vi "FPGA Main_4Modules.vi"() -> ()   [LabVIEW 2015]
doc: "This FPGA Main VI contains a control loop running in parallel with an RT watchdog loop.\n- The Control Loop performs control calculations on four input channels in parallel, and outputs the results to four output channels.\n- The RT Watchdog Loop checks for a periodic 'pet' from the RT Main VI to ensure communications between RT and FPGA are maintained."
uses:
  <vilib>/eio/EIONode/EIONode.xnode
  <vilib>/rvi/eio/common/nirviEmuTemplateMethod_errors.vi
  <vilib>/eio/EIOPropertyNode/EIOPropertyNode.xnode
  <vilib>/rvi/DataTransferAndStorage/Container/XNode/niFpgaContainer.xnode
  <vilib>/rvi/eio/common/nirviEmuTemplatePropertyGet_errors.vi
  <vilib>/rvi/eio/common/nirviEmuTemplatePropertyGet_noerrors.vi
  <vilib>/rvi/eio/common/nirviEmuTemplatePropertySet_errors.vi
  <vilib>/rvi/eio/common/nirviEmuTemplatePropertySet_noerrors.vi
  <vilib>/rvi/interface/RandomDataEmulation/nirviRandomDataFpgaReadWriteTemplate.vi
  <vilib>/LabVIEW Targets/FPGA/cRIO/shared/nicrio_ModuleControls/nicrio_cRIO-9234_DataRatesRing2.ctl
panel:
  in  "Data Rate":T1=1 items=["51.200 kS/s (NI 9234)"=1, "25.600 kS/s (NI 9234)"=2, "17.067 kS/s (NI 9234)"=3, "12.800 kS/s (NI 9234)"=4, "10.240 kS/s (NI 9234)"=5, "8.533 kS/s (NI 9234)"=6, "7.314 kS/s (NI 9234)"=7, "6.400 kS/s (NI 9234)"=8, "5.689 kS/s (NI 9234)"=9, "5.120 kS/s (NI 9234)"=10, "4.654 kS/s (NI 9234)"=11, "4.267 kS/s (NI 9234)"=12, "3.938 kS/s (NI 9234)"=13, "3.657 kS/s (NI 9234)"=14, "3.413 kS/s (NI 9234)"=15, "3.200 kS/s (NI 9234)"=16, "3.012 kS/s (NI 9234)"=17, "2.845 kS/s (NI 9234)"=18, "2.695 kS/s (NI 9234)"=19, "2.560 kS/s (NI 9234)"=20, "2.438 kS/s (NI 9234)"=21, "2.328 kS/s (NI 9234)"=22, "2.226 kS/s (NI 9234)"=23, "2.133 kS/s (NI 9234)"=24, "2.048 kS/s (NI 9234)"=25, "1.969 kS/s (NI 9234)"=26, "1.896 kS/s (NI 9234)"=27, "1.829 kS/s (NI 9234)"=28, "1.765 kS/s (NI 9234)"=29, "1.707 kS/s (NI 9234)"=30, "1.652 kS/s (NI 9234)"=31]
  out "FPGA Error":errorcluster
  out "Finished":bool
  in  "Stop":bool
  out "Module Underflow":bool
  out "DMA FIFO Full":bool
  out "Different Channel Count":bool
  out "Actual Loop Period (ticks)":u32
  out "First Read":bool
  in  "Number of Channels":i32=16
  in  "Channel Scale Array":fxp<+,24,12>[](array[numeric])=[0.0, 0.0, 0.0, 0.0, 0.0, 0.0, 0.0, 0.0, 0.0, 0.0, 0.0, 0.0, 0.0, 0.0, 0.0, 0.0]
  # "General Settings"
  # "Monitoring Values"
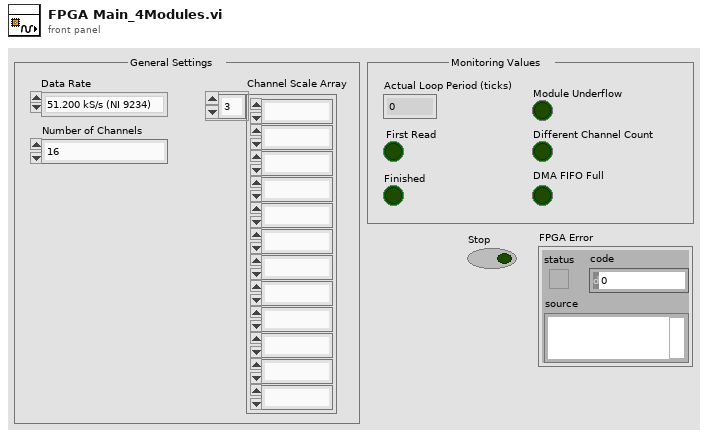
[diagram p1: front panel]
types:
  T1 = typedef "nicrio_cRIO-9234_DataRatesRing2.ctl" = u8
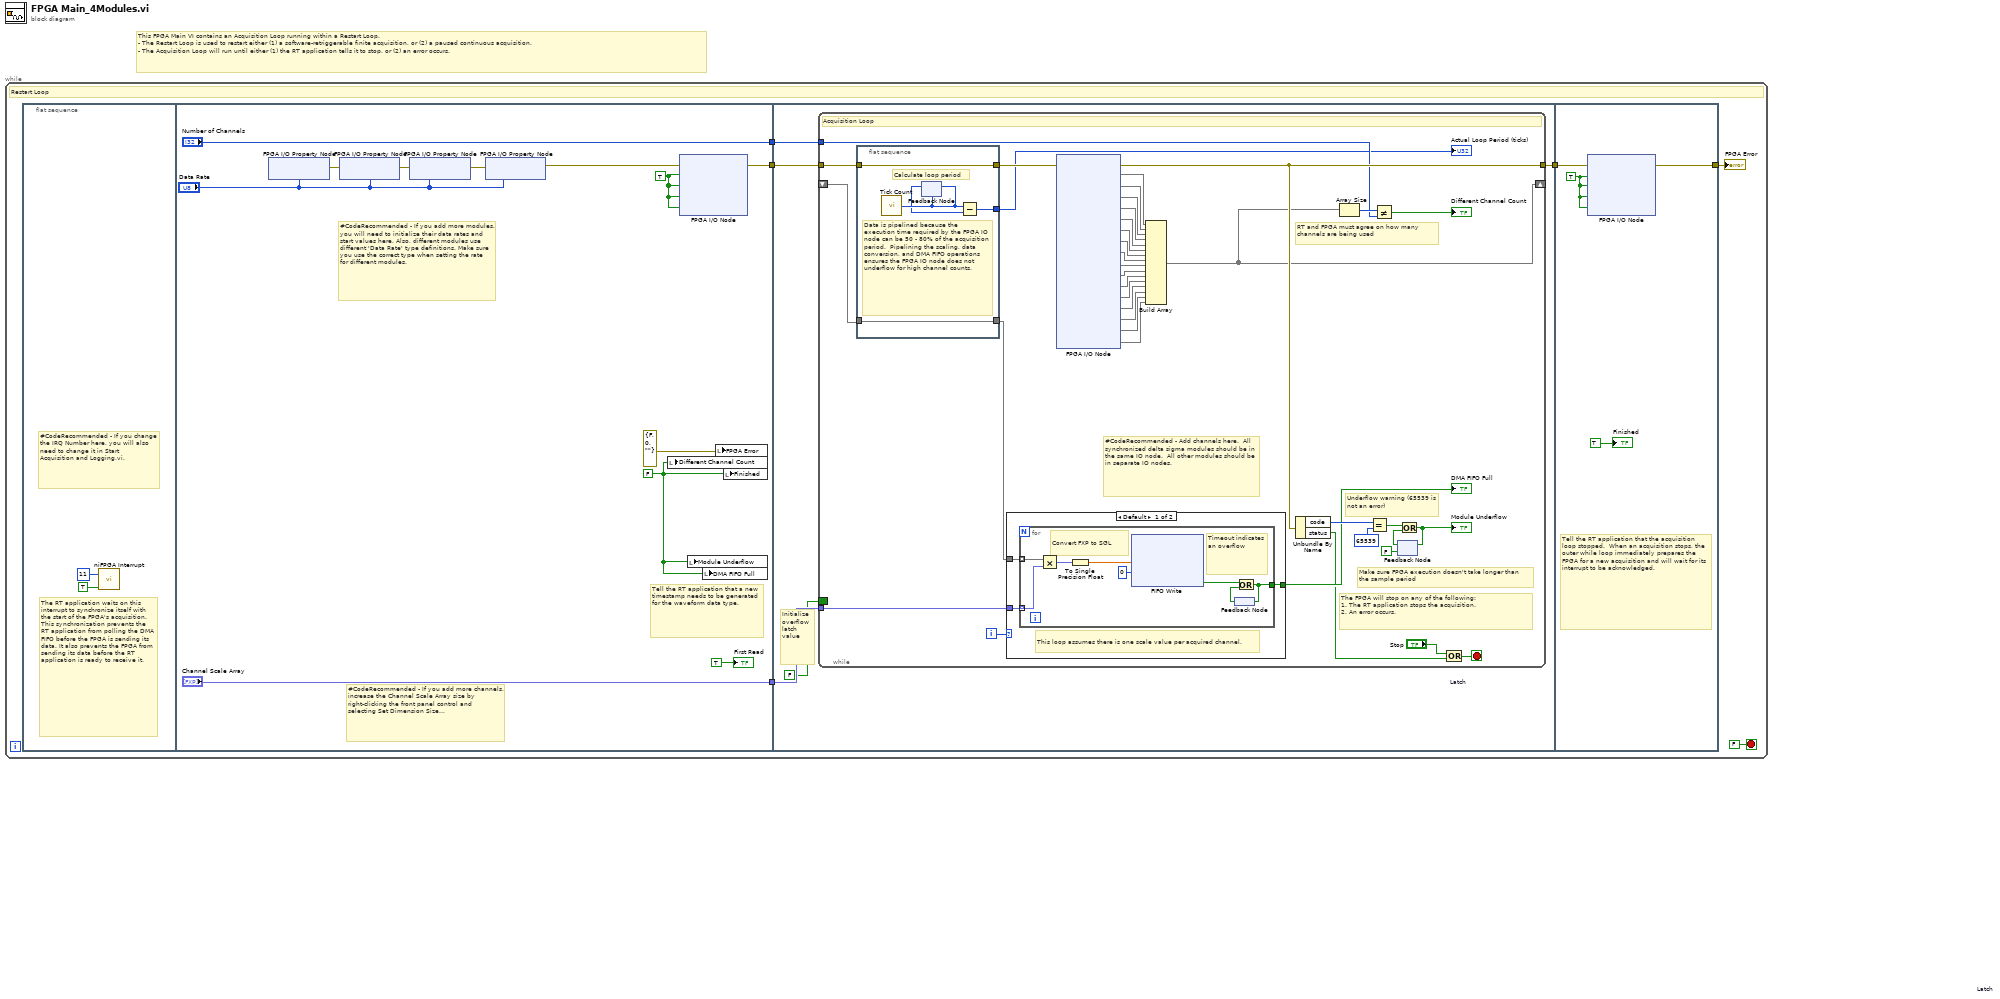
[diagram p0: block diagram]
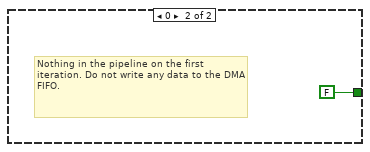
[diagram p2: hidden frame]
diagram:
  # "This FPGA Main VI contains an Acquisition Loop running within a Restart Loop.\n- The Restart Loop is used to restart either (1) a software-retriggerable finite acquisition, or (2) a paused continuous acquisition.\n- The Acquisition Loop will run until either (1) the RT application tells it to stop, or (2) an error occurs."
  n1 = while {
    stop <- FALSE stop-if-true
    # "Restart Loop"
    n2 = flat-sequence {
      tunnel: [w20] -> w5
      tunnel: ["Channel Scale Array"] -> w4
      tunnel: ["Number of Channels"] -> w3
      tunnel: w5 -> [w24]
      tunnel: w4 -> [w23]
      tunnel: w3 -> [w25]
      tunnel: [w22] -> w2
      tunnel: w2 -> [w83]
      tunnel: [w82] -> w1
      frame #0 {
        # "#CodeRecommended - If you change the IRQ Number here, you will also need to change it in Start Acquisition and Logging.vi."
        # "The RT application waits on this interrupt to synchronize itself with the start of the FPGA's acquisition.  This synchronization prevents the RT application from polling the DMA FIFO before the FPGA is sending its data. It also prevents the FPGA from sending its data before the RT application is ready to receive it."
        n3 = call <vilib>:"niFPGA Interrupt.vi"("Wait Until Cleared (F)"=TRUE ("Wait Until Cleared"), "IRQ Number (0)"=u8 11 ("IRQ Number")) -> ()  [unwired: 1 in]
      }
      frame #1 {
        w18 = FALSE ("Module Underflow")
        w9 = TRUE ("Mod1/Start")
        # "Tell the RT application that a new timestamp needs to be generated for the waveform data type."
        # "#CodeRecommended - If you add more channels, increase the Channel Scale Array size by right-clicking the front panel control and selecting Set Dimension Size..."
        # "#CodeRecommended - If you add more modules, you will need to initialize their data rates and start values here. Also, different modules use different 'Data Rate' type definitions. Make sure you use the correct type when setting the rate for different modules."
        n4 = xnode "FPGA I/O Property Node"("Data Rate"="Data Rate") -> ("error out"=w14:errorcluster)  [unwired: 2 in, 1 out]
        n5 = xnode "FPGA I/O Property Node"("error in"=w14, "Data Rate"="Data Rate") -> ("error out"=w12:errorcluster)  [unwired: 1 in, 1 out]
        n6 = xnode "FPGA I/O Property Node"("error in"=w12, "Data Rate"="Data Rate") -> ("error out"=w13:errorcluster)  [unwired: 1 in, 1 out]
        n7 = xnode "FPGA I/O Property Node"("error in"=w13, "Data Rate"="Data Rate") -> ("error out"=w10:errorcluster)  [unwired: 1 in, 1 out]
        n8 = local write "Different Channel Count"(w18) -> ()
        n9 = xnode "FPGA I/O Node"("error in"=w10, "Mod1/Start"=w9, "Mod2/Start"=w9, "Mod3/Start"=w9, "Mod4/Start"=w9) -> ("error out"=w20:errorcluster)  [unwired: 4 in, 4 out]
        n10 = local write "Module Underflow"(w18) -> ()
        n11 = local write "DMA FIFO Full"(w18) -> ()
        n12 = local write "FPGA Error"(errorcluster {"status"=FALSE, "code"=0, "source"=""} ("FPGA Error")) -> ()
        n13 = local write "Finished"(w18) -> ()
        "First Read" <- TRUE ("First Read")
      }
      frame #2 {
        # "Initialize overflow latch value"
        n14 = while {
          tunnel: w24 -> [w55]
          tunnel: [w60] -> w22
          shift-right: [w45] -> _
          shift-left: _ -> [w47]
          tunnel: w25 -> [w57]
          tunnel: w23 -> [w49]
          border: FALSE ("Overflow\nLatch") -> [_]
          i -> [w38]
          stop <- w63 stop-if-true
          # "Underflow warning (65539 is not an error)"
          # "The FPGA will stop on any of the following:\n1. The RT application stops the acquisition.\n2. An error occurs."
          # "#CodeRecommended - Add channels here.  All synchronized delta sigma modules should be in the same IO node.  All other modules should be in separate IO nodes."
          # "RT and FPGA must agree on how many channels are being used"
          # "Make sure FPGA execution doesn't take longer than the sample period"
          # "Acquisition Loop"
          n15 = flat-sequence {
            tunnel: [w80] -> w54
            tunnel: w55 -> [w80]
            tunnel: [w77] -> w53
            tunnel: w47 -> [w76]
            tunnel: [w76] -> w48
            frame #0 {
              # "Data is pipelined because the execution time required by the FPGA IO node can be 50 - 80% of the acquisition period.  Pipelining the scaling, data conversion, and DMA FIFO operations ensures the FPGA IO node does not underflow for high channel counts."
              # "Calculate loop period"
              n16 = call "Tick Count"() -> ("Tick Count(Ticks)"=w79:u32)
              n17 = feedback-in #1(w79) -> ()
              n18 = feedback #1(w79) -> (w78:u32)
              n19 = Subtract(x=w79, y=w78) -> (x-y=w77:u32)
            }
          }
          n20 = case shown="Default" w38 {
            tunnel: [w66 FALSE] -> w59
            tunnel: w49 -> [w65 _]
            tunnel: w48 -> [w64 _]
            frame Default {
              # "This loop assumes there is one scale value per acquired channel."
              n21 = for {
                tunnel: [w72] -> w66
                tunnel: w64 -> [w70] mode=indexing
                tunnel: w65 -> [w69] mode=indexing
                # "Timeout indicates an overflow"
                # "Convert FXP to SGL"
                n22 = Multiply(x=w70, y=w69) -> (x*y=w68:fxp<+,48,24>)
                n23 = To Single Precision Float(number=w68) -> (single precision float=w67:sgl)
                n24 = xnode ("FIFO Write")("Element"=w67, "Timeout"=0) -> ("Timed Out?"=w74:bool)  [unwired: 1 in, 1 out]
                n25 = feedback #2 "Latch"() -> (w73:bool)
                n26 = Or(x=w74, y=w73) -> (x .or. y?=w72:bool)
                n27 = feedback-in #2(w72) -> ()
              }
            }
            frame 0 {
              # "Nothing in the pipeline on the first iteration. Do not write any data to the DMA FIFO."
            }
          }
          "DMA FIFO Full" <- w59
          n28 = xnode "FPGA I/O Node"("error in"=w54) -> ("error out"=w60:errorcluster, "Mod1/AI0"=w52, "Mod1/AI1"=w46, "Mod1/AI2"=w51, "Mod1/AI3"=w50, "Mod2/AI0"=w37, "Mod2/AI1"=w36, "Mod2/AI2"=w35, "Mod2/AI3"=w34, "Mod3/AI0"=w33, "Mod3/AI1"=w32, "Mod3/AI2"=w31, "Mod3/AI3"=w30, "Mod4/AI0"=w29, "Mod4/AI1"=w28, "Mod4/AI2"=w27, "Mod4/AI3"=w26)  [unwired: 16 in, 16 out]
          n29 = Build Array(w52, w46, w51, w50, w37, w36, w35, w34, w33, w32, w31, w30, w29, w28, w27, w26) -> (w45:void[])
          n30 = Unbundle By Name(w60) -> ("code"=w61:i32, "status"=w40:bool)
          n31 = Array Size(array=w45) -> (size(s)=w58:i32)
          n32 = Equal?(x=w61, y=65539) -> (x = y?=w42:bool)
          n33 = Not Equal?(x=w58, y=w57) -> (x != y?=→"Different Channel Count":bool)
          n34 = feedback #3 "Latch"(FALSE) -> (w44:bool)
          n35 = Or(x=w42, y=w44) -> (x .or. y?=w41:bool)
          "Module Underflow" <- w41
          n36 = feedback-in #3(w41) -> ()
          n37 = Compound Arithmetic op=OR("Stop", w40) -> (w63:bool)
          "Actual Loop Period (ticks)" <- w53
        }
      }
      frame #3 {
        w81 = TRUE ("Mod1/Stop")
        # "Tell the RT application that the acquisition loop stopped.  When an acquisition stops, the outer while loop immediately prepares the FPGA for a new acquisition and will wait for its interrupt to be acknowledged."
        n38 = xnode "FPGA I/O Node"("error in"=w83, "Mod1/Stop"=w81, "Mod2/Stop"=w81, "Mod3/Stop"=w81, "Mod4/Stop"=w81) -> ("error out"=w82:errorcluster)  [unwired: 4 in, 4 out]
        "Finished" <- TRUE ("Finished")
      }
    }
    "FPGA Error" <- w1
  }
